vi "Undertake Check for New Command.vi"(8 "Current Command":T6, 10 "Wait time (ms)":dbl, 11 "Finished?":bool) -> (0 "Completion":T4, 1 "Subsystem Name":string, 2 "Current Command":T1, 3 "Initial Trace String":string, 4 "NextCommand":T6)   [LabVIEW 2023]
doc: "This VI is called for each controller loop iteration. It checks for new commands, updates timing data, and upon completion, notifies any waiting commands."
uses:
  Undertake Setpoints.ctl
  Undertake Operations.ctl
  <vilib>/Rock Robotics/WPI/Framework/Command Status Info.ctl
  <vilib>/Rock Robotics/WPI/Framework/Completion Status.ctl
  <vilib>/Rock Robotics/WPI/Framework/Completion Notifier.ctl
  Undertake Published Globals.vi
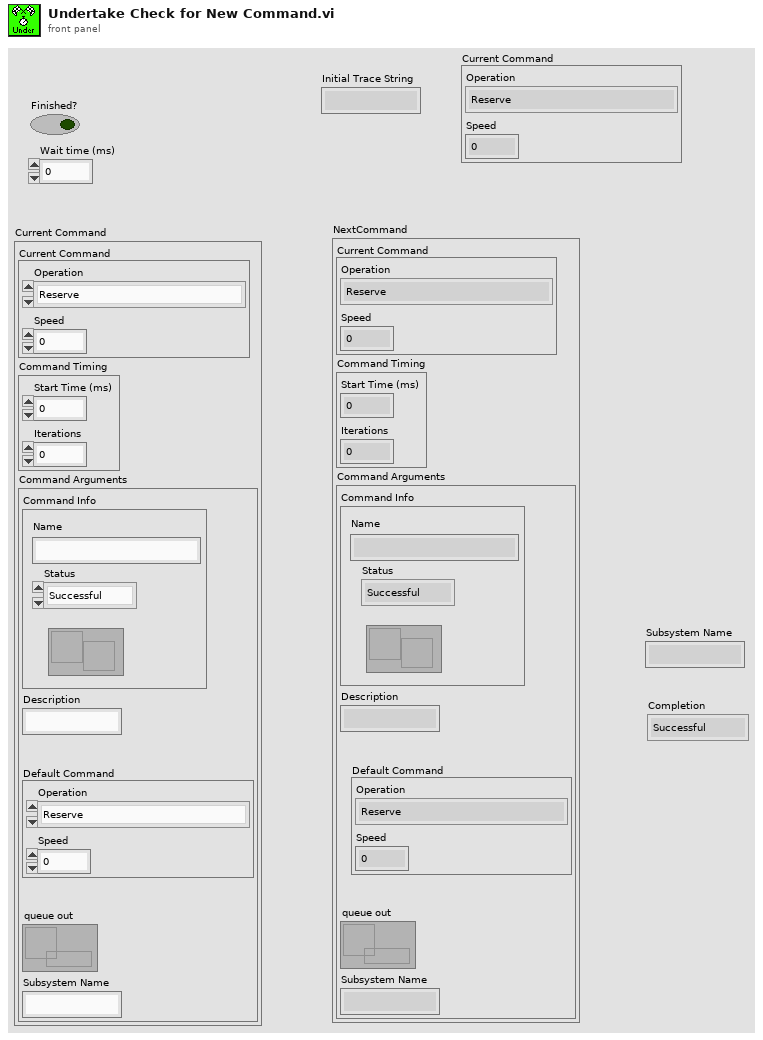
[diagram p1: front panel]
types:
  T1 = typedef "Undertake Setpoints.ctl" = cluster{"Operation":T2, "Speed":dbl}
  T2 = typedef "Undertake Operations.ctl" = enum16{"Reserve", "Read Current", "Immediate", "Onn", "Offf", "Reject"}
  T3 = typedef "Command Status Info.ctl" = cluster{"Name":string, "Status":T4, "notifier out":T5}
  T4 = typedef "Completion Status.ctl" = enum16{"Successful", "Aborted", "Incomplete"}
  T5 = typedef "Completion Notifier.ctl" = refnum<notifier>
  T6 = cluster{"Current Command":T1, "Command Timing":cluster{"Start Time (ms)":u32, "Iterations":i32}, "Command Arguments":cluster{"Command Info":T3, "Description":string, "Default Command":T1, "queue out":refnum<queue>, "Subsystem Name":string}}
  T7 = cluster{"Command Info":T3, "Description":string, "Default Command":T1, "queue out":refnum<queue>, "Subsystem Name":string}
  T8 = cluster{"Default Command":T1, "Command Info":T3, "Description":string}
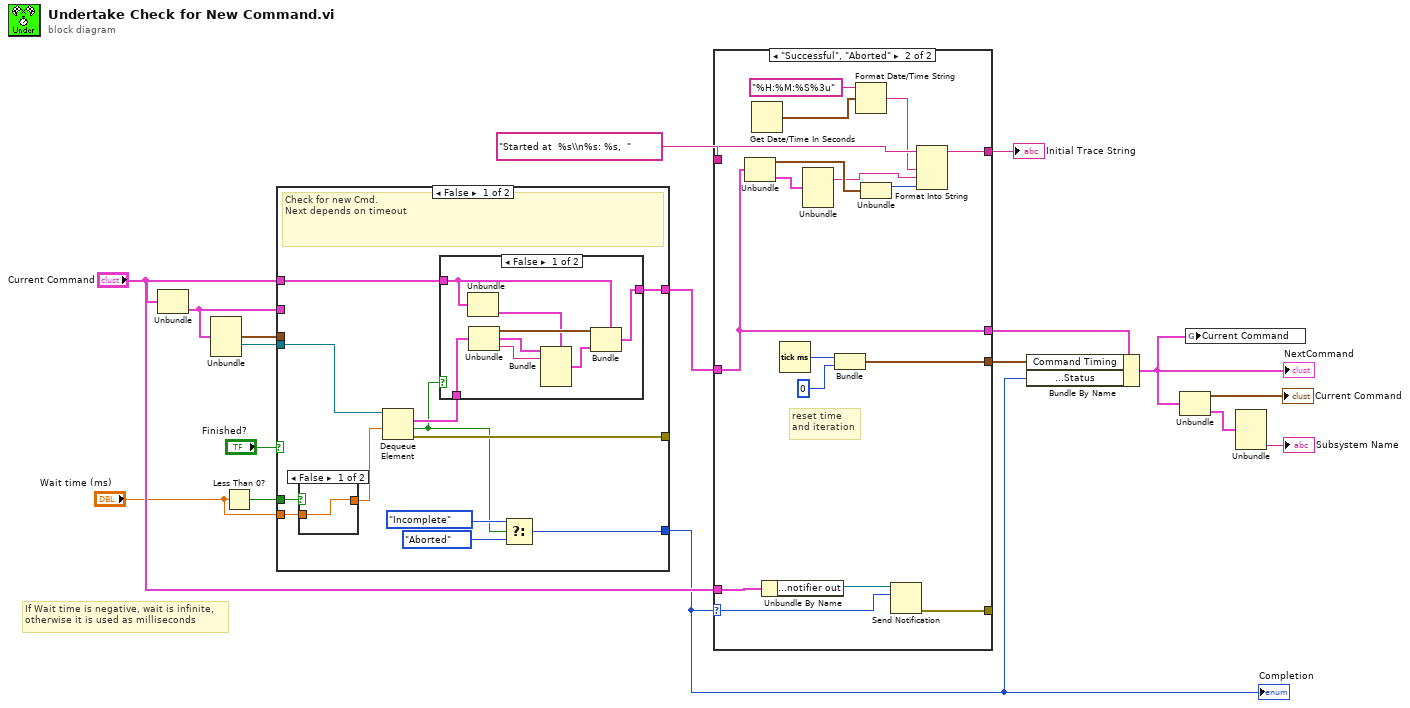
[diagram p0: block diagram]
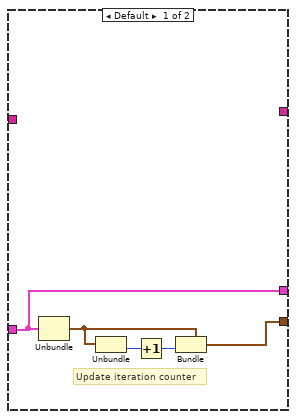
[diagram p2: hidden frame]
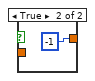
[diagram p4: hidden frame]
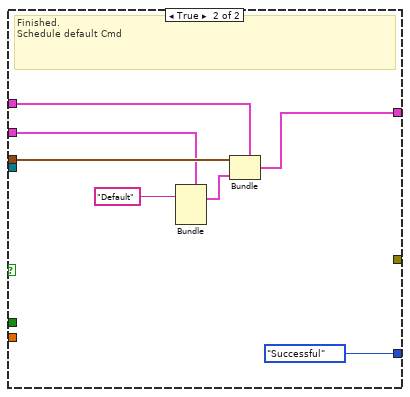
[diagram p5: hidden frame]
diagram:
  # "If Wait time is negative, wait is infinite,\notherwise it is used as milliseconds"
  n1 = Unbundle("Current Command") -> ("Command Arguments"=w7:T7)  [unwired: 2 out]
  n2 = Unbundle(w7) -> ("Default Command"=w10:T1, "queue out"=w11:refnum<queue>)  [unwired: 3 out]
  n3 = Less Than 0?(x="Wait time (ms)") -> (x < 0?=w6:bool)
  n4 = case shown="False" "Finished?" {
    tunnel: [w24 w46] -> w14
    tunnel: w6 -> [w26 _]
    tunnel: [w29 Completion_Status."Successful"] -> w1
    tunnel: [w21 _] -> _
    tunnel: w11 -> [w23 _]
    tunnel: "Current Command" -> [w25 w45]
    tunnel: w10 -> [_ w44]
    tunnel: w7 -> [_ w42]
    tunnel: "Wait time (ms)" -> [w18 _]
    frame False {
      # "Check for new Cmd.\nNext depends on timeout"
      n5 = case shown="False" w26 {
        tunnel: [w39 -1] -> w22
        tunnel: w18 -> [w39 _]
        frame False {
        }
        frame True {
        }
      }
      n6 = Dequeue Element(queue=w23, timeout in ms (-1)=w22) -> (element=w20:T8, timed out?=w19:bool, error out=w21:errorcluster)  [unwired: 1 in, 1 out]
      n7 = case shown="False" w19 {
        tunnel: w20 -> [w37 _]
        tunnel: w25 -> [w34 w38]
        tunnel: [w30 w38] -> w24
        frame False {
          n8 = Unbundle(w34) -> ("Command Arguments"=w33:T7)  [unwired: 2 out]
          n9 = Unbundle(w37) -> ("Default Command"=w36:T1, "Command Info"=w31:T3, "Description"=w32:string)
          n10 = Bundle(cluster=w33, "Command Info"=w31, "Description"=w32) -> (w35:T7)  [unwired: 3 in]
          n11 = Bundle(cluster=w34, "Current Command"=w36, "Command Arguments"=w35) -> (w30:T6)  [unwired: 1 in]
        }
        frame True {
        }
      }
      n12 = Select(t=Completion_Status."Incomplete", s=w19, f=Completion_Status."Aborted") -> (s? t:f=w29:T4)
    }
    frame True {
      # "Finished.\nSchedule default Cmd"
      n13 = Bundle(cluster=w42, "Description"="Default") -> (w43:T7)  [unwired: 4 in]
      n14 = Bundle(cluster=w45, "Current Command"=w44, "Command Arguments"=w43) -> (w46:T6)  [unwired: 1 in]
    }
  }
  "Completion" <- w1
  n15 = case shown="\"Successful\", \"Aborted\"" w1 {
    selector: w1 -> [_ w69]
    tunnel: "Current Command" -> [_ w66]
    tunnel: "Started at  %s\\n%s: %s,  " ("format string") -> [_ w65]
    tunnel: [_ w64] -> w16
    tunnel: w14 -> [w49 w54]
    tunnel: [w48 w53] -> w2
    tunnel: [_ w59] -> _
    tunnel: [w49 w54] -> w3
    frame Default {
      # "Update iteration counter"
      n16 = Unbundle(w49) -> ("Command Timing"=w50:cluster{"Start Time (ms)":u32, "Iterations":i32})  [unwired: 2 out]
      n17 = Unbundle(w50) -> ("Iterations"=w51:i32)  [unwired: 1 out]
      n18 = Increment(x=w51) -> (x+1=w52:i32)
      n19 = Bundle(cluster=w50, "Iterations"=w52) -> (w48:cluster{"Start Time (ms)":u32, "Iterations":i32})  [unwired: 1 in]
    }
    frame "Successful", "Aborted" {
      # "reset time\nand iteration"
      n20 = Unbundle(w54) -> ("Current Command"=w63:T1, "Command Arguments"=w60:T7)  [unwired: 1 out]
      n21 = Get Date/Time In Seconds() -> (seconds since 1Jan1904=w58:timestamp)
      n22 = Unbundle By Name(w66) -> ("Command Arguments.Command Info.notifier out"=w68:T5)
      n23 = Tick Count (ms)() -> (millisecond timer value=w62:u32)
      n24 = Unbundle(w60) -> ("Description"=w57:string)  [unwired: 4 out]
      n25 = Bundle("millisecond timer value"=w62, 0) -> (w53:cluster{"millisecond timer value":u32, i32})  [unwired: 1 in]
      n26 = Format Date/Time String(time format string (%c)="%H:%M:%S%3u", seconds (now)=w58) -> (date/time string=w56:string)  [unwired: 1 in]
      n27 = Unbundle(w63) -> ("Operation"=w67:T2)  [unwired: 1 out]
      n28 = Send Notification(notification=w69, notifier=w68) -> (error out=w59:errorcluster)  [unwired: 1 in, 1 out]
      n29 = Format Into String(format string=w65, w56, w57, w67) -> (resulting string=w64:string)  [unwired: 2 in, 1 out]
    }
  }
  "Initial Trace String" <- w16
  n30 = Bundle By Name(cluster=w3, "Command Timing"=w2, "Command Arguments.Command Info.Status"=w1) -> (w4:T6)
  "NextCommand" <- w4
  n31 = Unbundle(w4) -> ("Current Command"=→"Current Command":T1, "Command Arguments"=w9:T7)  [unwired: 1 out]
  n32 = global write "Undertake Published Globals.vi" "Current Command"(w4) -> ()
  n33 = Unbundle(w9) -> ("Subsystem Name"=→"Subsystem Name":string)  [unwired: 4 out]
